vi "Initialise.vi"(8 "error in (no error)":errorcluster, 11 "PWM in":refnum<class "LINX-PCA9685 PWM.lvclass">) -> (0 "error out":errorcluster, 3 "PWM out":refnum<class "LINX-PCA9685 PWM.lvclass">)   [LabVIEW 2020, in "LINX-PCA9685 PWM.lvclass"]
doc: "Initialises the device with basic default values."
uses:
  LINX-PCA9685 PWM.lvclass
  LINX I2C/LINX I2C.lvclass
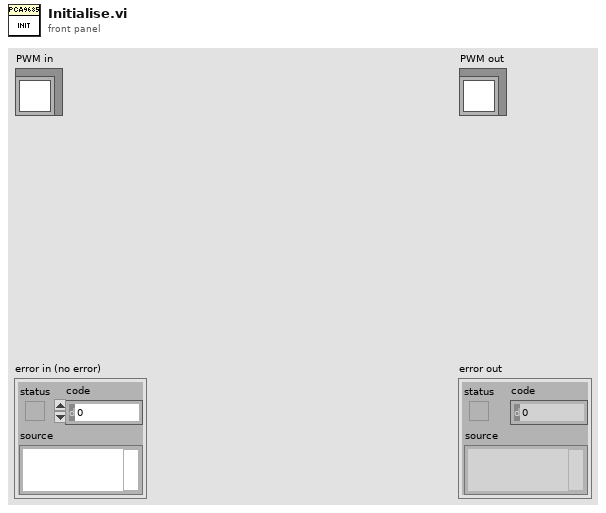
[diagram p1: front panel]
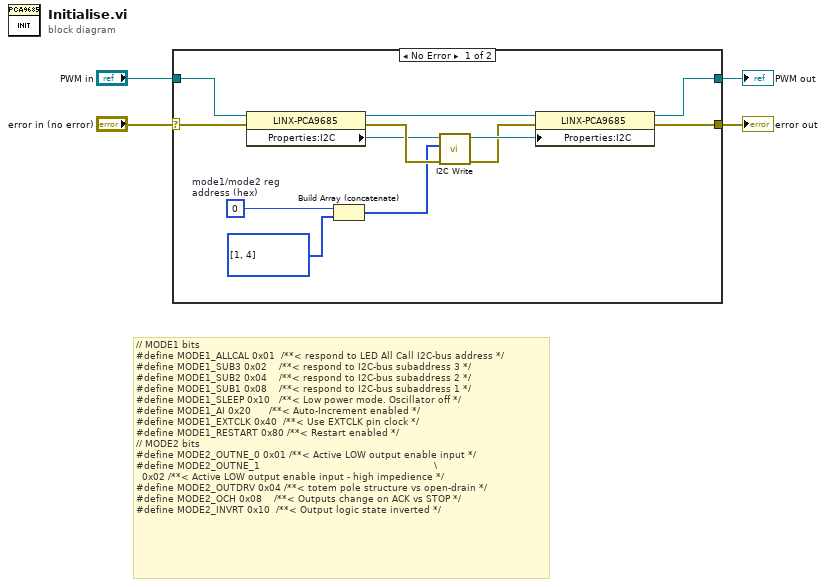
[diagram p0: block diagram]
diagram:
  # "// MODE1 bits\n#define MODE1_ALLCAL 0x01  /**< respond to LED All Call I2C-bus address */\n#define MODE1_SUB3 0x02    /**< respond to I2C-bus subaddress 3 */\n#define MODE1_SUB2 0x04    /**< respond to I2C-bus subaddress 2 */\n#define MODE1_SUB1 0x08    /**< respond to I2C-bus subaddress 1 */\n#define MODE1_SLEEP 0x10   /**< Low power mode. Oscillator off */\n#define MODE1_AI 0x20      /**< Auto-Increment enabled */\n#define MODE1_EXTCLK 0x40  /**< Use EXTCLK pin clock */\n#define MODE1_RESTART 0x80 /**< Restart enabled */\n// MODE2 bits\n#define MODE2_OUTNE_0 0x01 /**< Active LOW output enable input */\n#define MODE2_OUTNE_1                                                          \\\n  0x02 /**< Active LOW output enable input - high impedience */\n#define MODE2_OUTDRV 0x04 /**< totem pole structure vs open-drain */\n#define MODE2_OCH 0x08    /**< Outputs change on ACK vs STOP */\n#define MODE2_INVRT 0x10  /**< Output logic state inverted */"
  n1 = case shown="No Error" "error in (no error)" {
    selector: "error in (no error)" -> [w16 w18]
    tunnel: [w6 w18] -> w3
    tunnel: [w7 w17] -> w1
    tunnel: "PWM in" -> [w12 w17]
    frame No Error {
      w14 = u8 0  # mode1/mode2 reg address (hex)
      n2 = property class="LINX-PCA9685"(reference=w12, error in=w16) -> (reference out=w9:refnum<class "LINX-PCA9685 PWM.lvclass">, error out=w13:errorcluster, "Properties:I2C"=w11:refnum<class "LINX I2C.lvclass">)
      n3 = Build Array (concatenate)(w14, u8[] [1, 4] ("Data")) -> (w5:u8[])
      n4 = call "I2C Write.vi"("error in (no error)"=w13, "Bytes to Write"=w5, "LINX I2C in"=w11) -> ("error out"=w8:errorcluster, "LINX I2C out"=w10:refnum<class "LINX I2C.lvclass">)  [unwired: 7 in]
      n5 = property class="LINX-PCA9685"(reference=w9, error in=w8, "Properties:I2C"=w10) -> (reference out=w7:refnum<class "LINX-PCA9685 PWM.lvclass">, error out=w6:errorcluster)
    }
    frame Error {
    }
  }
  "error out" <- w3
  "PWM out" <- w1
